vi "Result Queue Ref FGV.vi"(6 "Q FGV":T1, 8 "error in":errorcluster, 11 "Set Queue":refnum<queue>) -> (0 "error out":errorcluster, 3 "Get Queue":refnum<queue>)   [LabVIEW 2023, in "HardwareAbstractionLayer_LVOOP.lvlib" / "Report.lvclass"]
uses:
  Report.lvclass
  Control/Queue FGV.ctl
  Control/Q Data.ctl
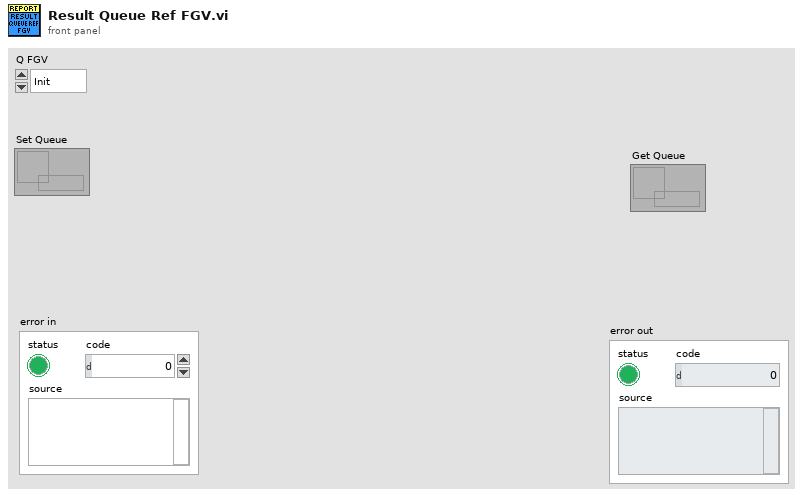
[diagram p1: front panel]
types:
  T1 = typedef "HardwareAbstractionLayer_LVOOP.lvlib/Report.lvclass/Queue FGV.ctl" = enum16{"Init", "Set", "Get"}
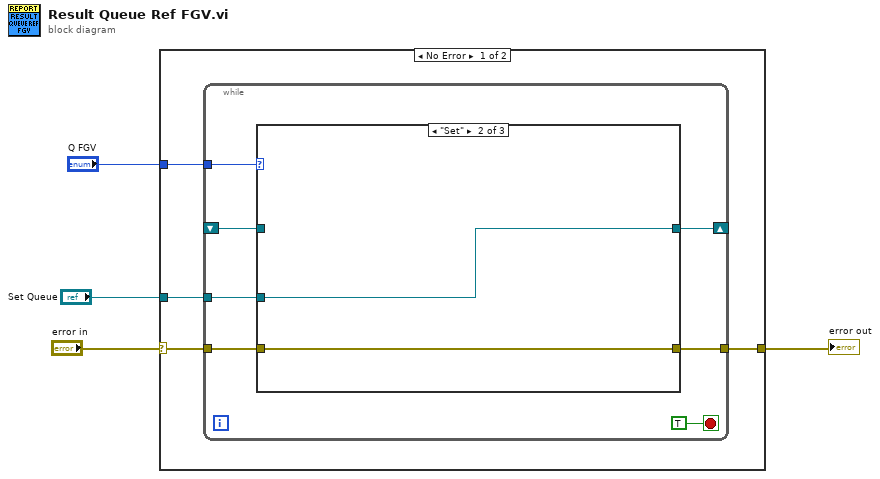
[diagram p0: block diagram]
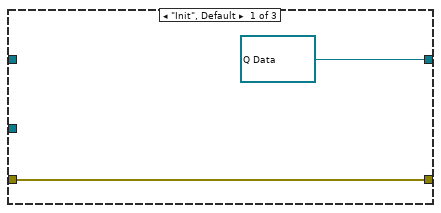
[diagram p2: hidden frame]
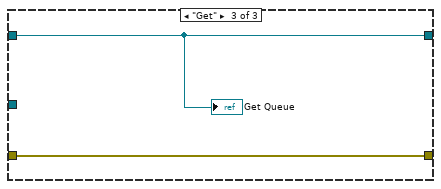
[diagram p3: hidden frame]
diagram:
  n1 = case shown="No Error" "error in" {
    selector: "error in" -> [w8 w22]
    tunnel: [w7 w22] -> w3
    tunnel: "Q FGV" -> [w6 _]
    tunnel: "Set Queue" -> [w5 _]
    frame No Error {
      n2 = while {
        tunnel: w8 -> [w14]
        tunnel: [w13] -> w7
        tunnel: w6 -> [w12]
        shift-right: [w11] -> _
        shift-left: _ -> [w9]
        tunnel: w5 -> [w10]
        stop <- TRUE stop-if-true
        n3 = case shown="\"Set\"" w12 {
          tunnel: w14 -> [w16 w19 w20]
          tunnel: [w16 w19 w20] -> w13
          tunnel: [refnum<queue> refnum ("queue out") w18 w21] -> w11
          tunnel: w10 -> [_ w18 _]
          tunnel: w9 -> [_ _ w21]
          frame "Init", Default {
          }
          frame "Set" {
          }
          frame "Get" {
            "Get Queue" <- w21
          }
        }
      }
    }
    frame Error {
    }
  }
  "error out" <- w3
